vi "LaunchDragItem.vi"(8 "error in (no error)":errorcluster, 11 "OrderSelection in":refnum<class "OrderSelection.lvclass">) -> (0 "error out":errorcluster, 3 "OrderSelection out":refnum<class "OrderSelection.lvclass">)   [LabVIEW 2015, in "OrderSelection.lvclass"]
uses:
  OrderSelection.lvclass
  DragItem.vi
  MouseUpCapture.vi
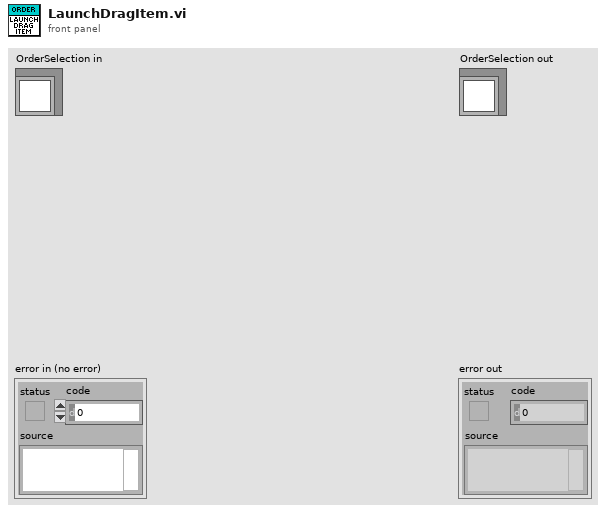
[diagram p1: front panel]
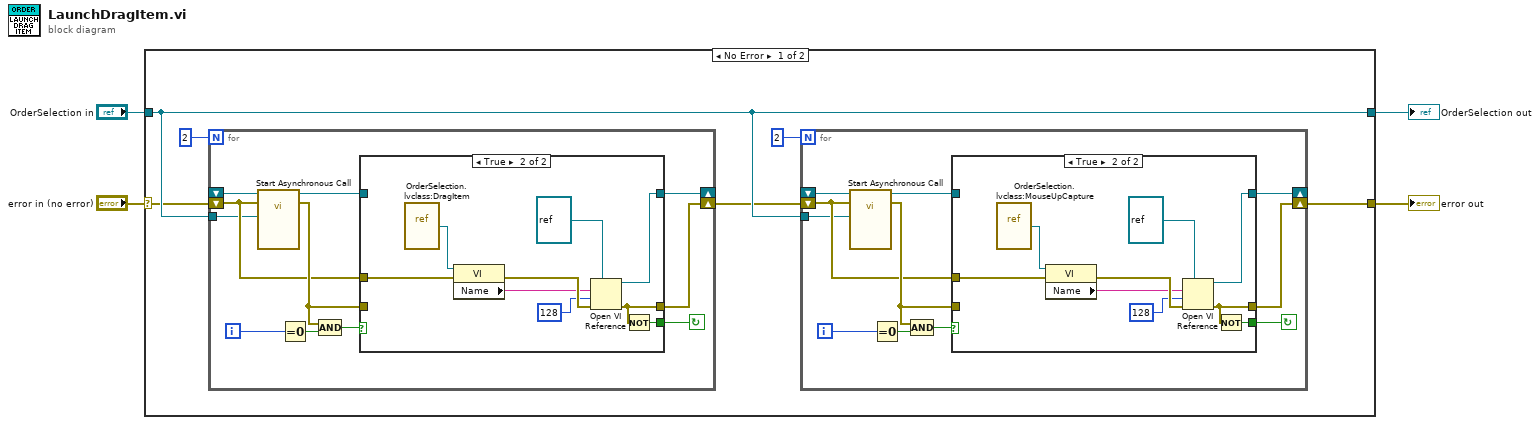
[diagram p0: block diagram]
diagram:
  n1 = case shown="No Error" "error in (no error)" {
    selector: "error in (no error)" -> [w5 w56]
    tunnel: [w9 w56] -> w3
    tunnel: [w7 w55] -> w1
    tunnel: "OrderSelection in" -> [w7 w55]
    frame No Error {
      n2 = for {
        N: 2 -> [_]
        shift-right: [w21] -> _
        shift-left: _ -> [w20]
        shift-right: [w18] -> w6
        shift-left: w5 -> [w12]
        tunnel: w7 -> [w11]
        i -> [w15]
        stop <- w13 continue-if-true
        n3 = call-by-ref "Start Asynchronous Call"(reference=w20, error in=w12, "OrderSelection in"=w11) -> (reference out=w19:refnum<vi>, error out=w14:errorcluster)  [unwired: 9 in, 2 out]
        n4 = Equal To 0?(x=w15) -> (x = 0?=w16:bool)
        n5 = Compound Arithmetic op=AND(w14, w16) -> (w17:bool)
        n6 = case shown="True" w17 {
          tunnel: [w23 w29] -> w21
          tunnel: [w22 w27] -> w18
          tunnel: w19 -> [w23 _]
          tunnel: w14 -> [w22 _]
          tunnel: [_ w28] -> w13
          tunnel: w12 -> [_ w26]
          frame False {
          }
          frame True {
            n7 = vi-ref "OrderSelection.lvclass:DragItem.vi"() -> (w25:refnum<vi>)
            n8 = property class="VI"(reference=w25, error in=w26) -> (error out=w32:errorcluster, "Name"=w31:string)  [unwired: 1 out]
            n9 = Open VI Reference(type specifier VI Refnum (for type only)=refnum<vi> refnum, vi path=w31, options=128, error in (no error)=w32) -> (vi reference=w29:refnum<vi>, error out=w27:errorcluster)  [unwired: 2 in]
            n10 = Not(x=w27) -> (.not. x?=w28:bool)
          }
        }
      }
      n11 = for {
        N: 2 -> [_]
        shift-right: [w43] -> _
        shift-left: _ -> [w42]
        shift-right: [w40] -> w9
        shift-left: w6 -> [w34]
        tunnel: w7 -> [w33]
        i -> [w37]
        stop <- w35 continue-if-true
        n12 = call-by-ref "Start Asynchronous Call"(reference=w42, error in=w34, "OrderSelection in"=w33) -> (reference out=w41:refnum<vi>, error out=w36:errorcluster)  [unwired: 10 in, 1 out]
        n13 = Equal To 0?(x=w37) -> (x = 0?=w38:bool)
        n14 = Compound Arithmetic op=AND(w36, w38) -> (w39:bool)
        n15 = case shown="True" w39 {
          tunnel: [w45 w51] -> w43
          tunnel: [w44 w49] -> w40
          tunnel: w41 -> [w45 _]
          tunnel: w36 -> [w44 _]
          tunnel: [_ w50] -> w35
          tunnel: w34 -> [_ w48]
          frame False {
          }
          frame True {
            n16 = vi-ref "OrderSelection.lvclass:MouseUpCapture.vi"() -> (w47:refnum<vi>)
            n17 = property class="VI"(reference=w47, error in=w48) -> (error out=w54:errorcluster, "Name"=w53:string)  [unwired: 1 out]
            n18 = Open VI Reference(type specifier VI Refnum (for type only)=refnum<vi> refnum, vi path=w53, options=128, error in (no error)=w54) -> (vi reference=w51:refnum<vi>, error out=w49:errorcluster)  [unwired: 2 in]
            n19 = Not(x=w49) -> (.not. x?=w50:bool)
          }
        }
      }
    }
    frame Error {
    }
  }
  "error out" <- w3
  "OrderSelection out" <- w1
